vi "get.vi"(8 "error in (no error)":errorcluster caption="错误输入（无错误）", 11 "HttpClient输入":refnum<class "Http.lvclass">) -> (0 "error out":errorcluster caption="错误输出", 2 "Url":string, 3 "HttpClient输出":refnum<class "Http.lvclass">)   [LabVIEW 2012, in "Http.lvclass"]
uses:
  Http.lvclass
  Http.lvclass/Http.ctl
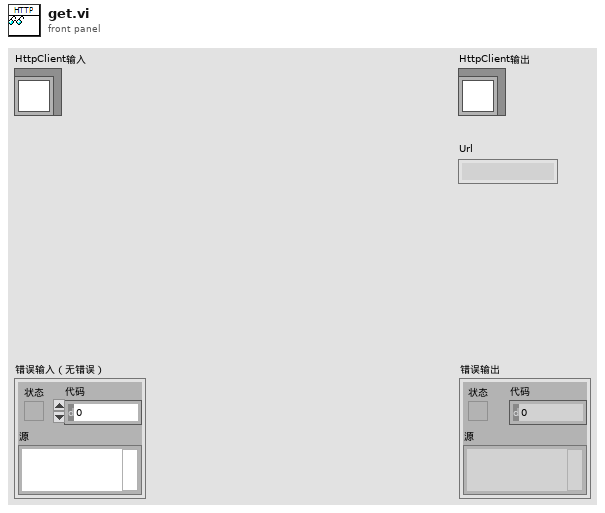
[diagram p1: front panel]
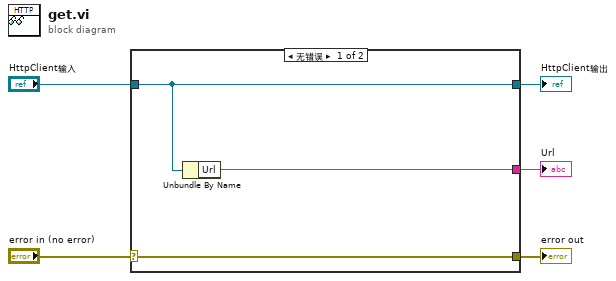
[diagram p0: block diagram]
diagram:
  n1 = case shown="无错误" "error in (no error)" {
    selector: "error in (no error)" -> [w8 w9]
    tunnel: [w8 w9] -> w4
    tunnel: [w7 w10] -> w2
    tunnel: "HttpClient输入" -> [w7 w10]
    tunnel: [w6 _] -> w1
    frame No Error {
      n2 = Unbundle By Name(w7) -> ("Url"=w6:string)
    }
    frame Error {
    }
  }
  "error out" <- w4
  "HttpClient输出" <- w2
  "Url" <- w1
